vi "Write Action settings.vi"(8 "error in (no error)":errorcluster, 10 "Action settings":T1, 11 "Motor in":refnum<class "Motor.lvclass">) -> (0 "error out":errorcluster, 3 "Motor out":refnum<class "Motor.lvclass">)   [LabVIEW 2013, in "PowderDeposition.lvlib" / "Motor.lvclass"]
uses:
  Motor.lvclass
  Action-settings.ctl
  Motor.lvclass/Motor.ctl
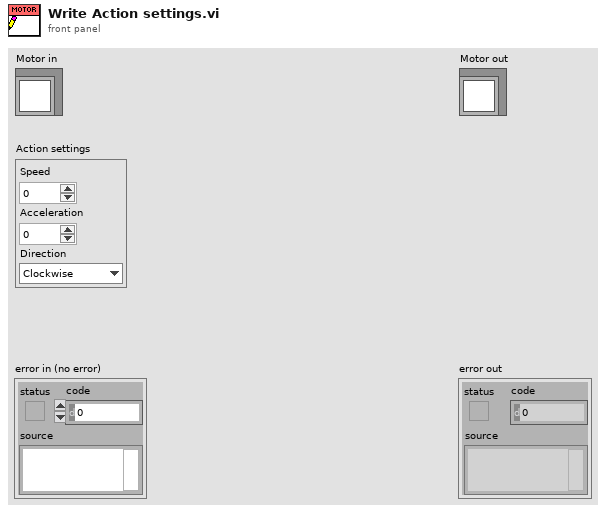
[diagram p1: front panel]
types:
  T1 = typedef "PowderDeposition.lvlib/Motor.lvclass/Action-settings.ctl" = cluster{"Speed":dbl, "Acceleration":dbl, "Direction":enum16{"Clockwise", "Counter-clockwise"}}
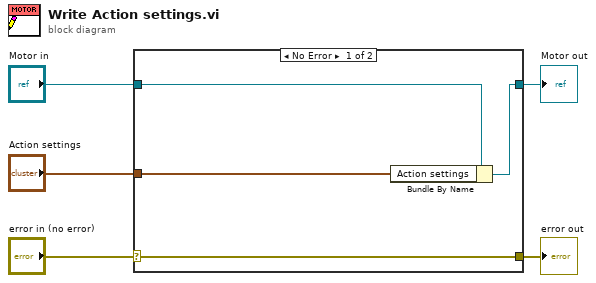
[diagram p0: block diagram]
diagram:
  n1 = case shown="No Error" "error in (no error)" {
    selector: "error in (no error)" -> [w9 w10]
    tunnel: [w9 w10] -> w4
    tunnel: [w7 w11] -> w2
    tunnel: "Motor in" -> [w8 w11]
    tunnel: "Action settings" -> [w6 _]
    frame No Error {
      n2 = Bundle By Name(cluster=w8, "Action settings"=w6) -> (w7:refnum<class "Motor.lvclass">)
    }
    frame Error {
    }
  }
  "error out" <- w4
  "Motor out" <- w2
